vi "Constants.vi"() -> ()   [LabVIEW 2019, in "TemplatePPL Shared.lvlib"]
doc: "Use this Global VI to access the GUIDs assigned to the page resources of the Custom Device."
uses:
  TemplatePPL Shared.lvlib
panel:
  in  "Tab Control":enum32{"GUIDs", "Constants", "Properties"}(tab)
  in  "ExtraPage3":string="ed223695-9742-4212-80b8-e36db0930e33"
  in  "ExtraPage2":string="63d35a8b-3e35-4a3c-929e-a7d8420c2430"
  in  "ExtraPage1":string="6d6e2c98-ce83-442d-aecf-42009e8827cd"
  in  "TemplatePPL":string="136665a4-4318-4fea-b2af-48bf65c2c90e"
  in  "Compiled.Settings":string="Compiled.Settings"
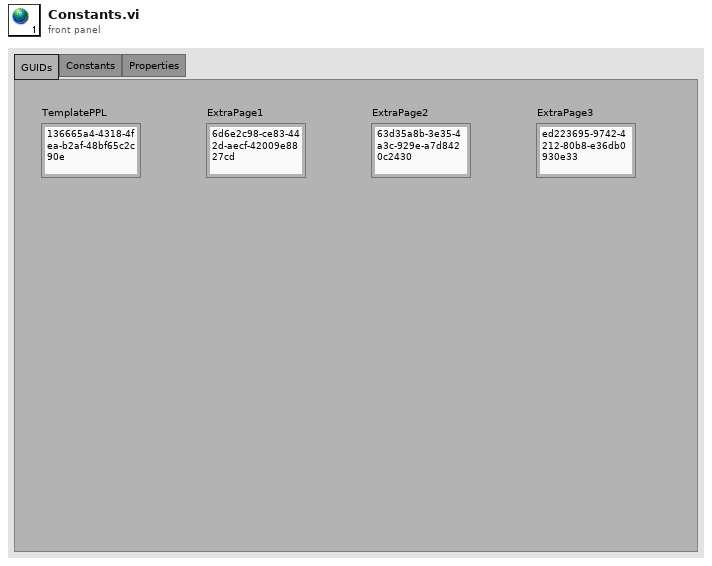
[diagram p1: front panel]
diagram:
